vi "Init HTTP.vi"(8 "error in (no error)":errorcluster, 11 "Log Manager Module in":refnum<class "Log Manager Module.lvclass">) -> (0 "error out":errorcluster, 3 "Log Manager Module out":refnum<class "Log Manager Module.lvclass">)   [LabVIEW 2020, in "VolatusData.lvlib" / "Log Manager Module.lvclass"]
uses:
  Log Manager Module.lvclass
  Log Manager Module.lvclass/Log Manager Module.ctl
  Volatus/Module/Module.lvclass
  Volatus/VolatusAPI/VolatusAPI.lvclass
  LogHTTPController/LogHTTPController.lvclass
  C:/dev/lv20CE/relink/lv-volatus/Volatus/Module/Module.lvclass
  C:/dev/lv20CE/relink/lv-volatus/VolatusData/Log Manager Module/Log Manager Module.lvclass
  C:/dev/lv20CE/relink/lv-http-server/HTTP Server/Controller/Controller.lvclass
  C:/dev/lv20CE/relink/lv-http-server/HTTP Server/Handler/Handler.lvclass
  C:/dev/lv20CE/relink/lv-volatus/VolatusData/LogHTTPController/LogHTTPController.lvclass
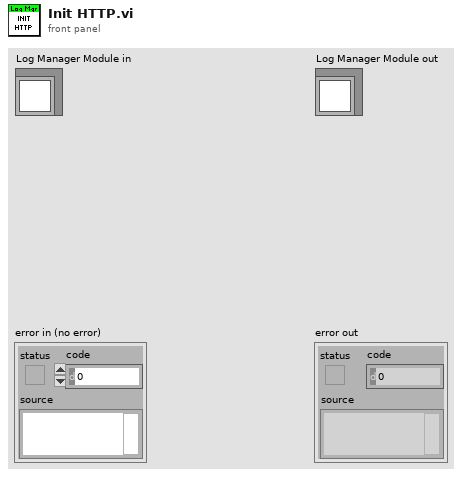
[diagram p1: front panel]
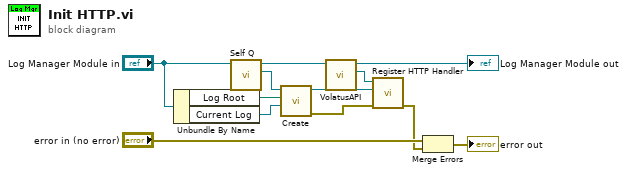
[diagram p0: block diagram]
diagram:
  n1 = Unbundle By Name("Log Manager Module in") -> ("Log Root"=w6:path, "Current Log"=w5:refnum<notifier>)
  n2 = call "Self Q.vi"("Module in"="Log Manager Module in") -> ("Self Q"=w7:refnum<class "MessageQ.lvclass">, "Module out"=w8:refnum<class "Log Manager Module.lvclass">)  [unwired: 9 in]
  n3 = call "Create.vi"("Current Log"=w5, "Log Folder"=w6, "LogManager"=w7) -> ("error out"=w3:errorcluster, "LogHTTPController out"=w4:refnum<class "LogHTTPController.lvclass">)  [unwired: 7 in]
  n4 = call "VolatusAPI.vi"("Module in"=w8) -> ("VolatusAPI"=w10:refnum<class "VolatusAPI.lvclass">, "Module out"=→"Log Manager Module out":refnum<class "Log Manager Module.lvclass">)  [unwired: 9 in]
  n5 = call "Register HTTP Handler.vi"("error in (no error)"=w3, "Handler"=w4, "VolatusAPI in"=w10) -> ("error out"=w1:errorcluster)  [unwired: 7 in, 1 out]
  n6 = Merge Errors("error in (no error)", w1) -> (→"error out":errorcluster)
